vi "Measurement UI.vi"() -> ()   [LabVIEW 2021, in "Efficiency And Load Regulation_PMIC.lvlib"]
uses:
  Efficiency And Load Regulation_PMIC.lvlib
panel:
  in  "MeasGraphs":T1(tab)
  out "EfficiencyGraph":T2(graph)
  out "LoadRegulationGraph(V/A)":T2(graph)
  out "LoadRegulationGraph(%)":T2(graph)
  out "Maximum load regulation":dbl[](array[numeric])
  out "Minimum load regulation":dbl[](array[numeric])
  out "Maximum load voltage":dbl[](array[numeric])
  out "Minimum load voltage":dbl[](array[numeric])
  out "Maximum efficiency":dbl[](array[numeric])
  out "Minimum efficiency":dbl[](array[numeric])
  out "Source sweep points":i32
  out "Load voltage deviation":dbl[](array[numeric])
  out "Load voltages":dbl[](array[numeric])
  out "Voltage values":dbl[](array[numeric])
  out "Load sweep points":i32
  out "Efficiency":dbl[](array[numeric])
  out "Load currents":dbl[](array[numeric])
  in  "Source resource name":string caption="RESOURCE NAME"
  in  "Load resource name":string caption="RESOURCE NAME"
  out "MeasTable":string[][](table)
  out "Status":string
  in  "ELOADResourceName":refnum<k15> caption="RESOURCE NAME"
  in  "PPSResourceName":refnum<k15> caption="RESOURCE NAME"
  in  "Load sweep type":string(combo)="Logarithmic" caption="SWEEP TYPE"
  in  "DUT setup time":dbl=1.0 caption="DUT SETUP TIME" format="%#_6ps"
  in  "Source stop voltage":dbl=20.0 caption="STOP VOLTAGE" format="%#_6pV"
  in  "Source start voltage":dbl=6.0 caption="START VOLTAGE" format="%#_6pV"
  in  "Source voltage sweep points":i32=4 caption="NO. OF POINTS"
  in  "Aperture time":dbl=0.005 caption="APERTURE TIME" format="%#_6ps"
  in  "Source delay":dbl=0.005 caption="SOURCE DELAY" format="%#_6ps"
  in  "Load current sweep points/points per decade":i32=10 caption="PTS/PTS PER DECADE"
  in  "Load stop current":dbl=24.0 caption="STOP CURRENT" format="%#_6pA"
  in  "Load start current":dbl=0.1 caption="START CURRENT" format="%#_6pA"
  in  "Load voltage limit range":dbl=6.0 caption="VOLTAGE LIMIT RANGE" format="%#_6pV"
  in  "Source current limit":dbl=25.0 caption="CURRENT LIMIT" format="%#_6pA"
  in  "Source maximum power":dbl=300.0 caption="MAXIMUM POWER" format="%#_6pW"
  in  "Load configuration":string="Load configuration"
  in  "Source configuration":string="Source configuration"
  in  "Measurement settings":string="Measurement settings"
  in  "Nominal output voltage":dbl=3.3 caption="NOMINAL OUTPUT VOLTAGE" format="%#_6pV"
  in  "Mode of operation":T3(ring)=enum."Perform measurement" caption="MODE OF OPERATION"
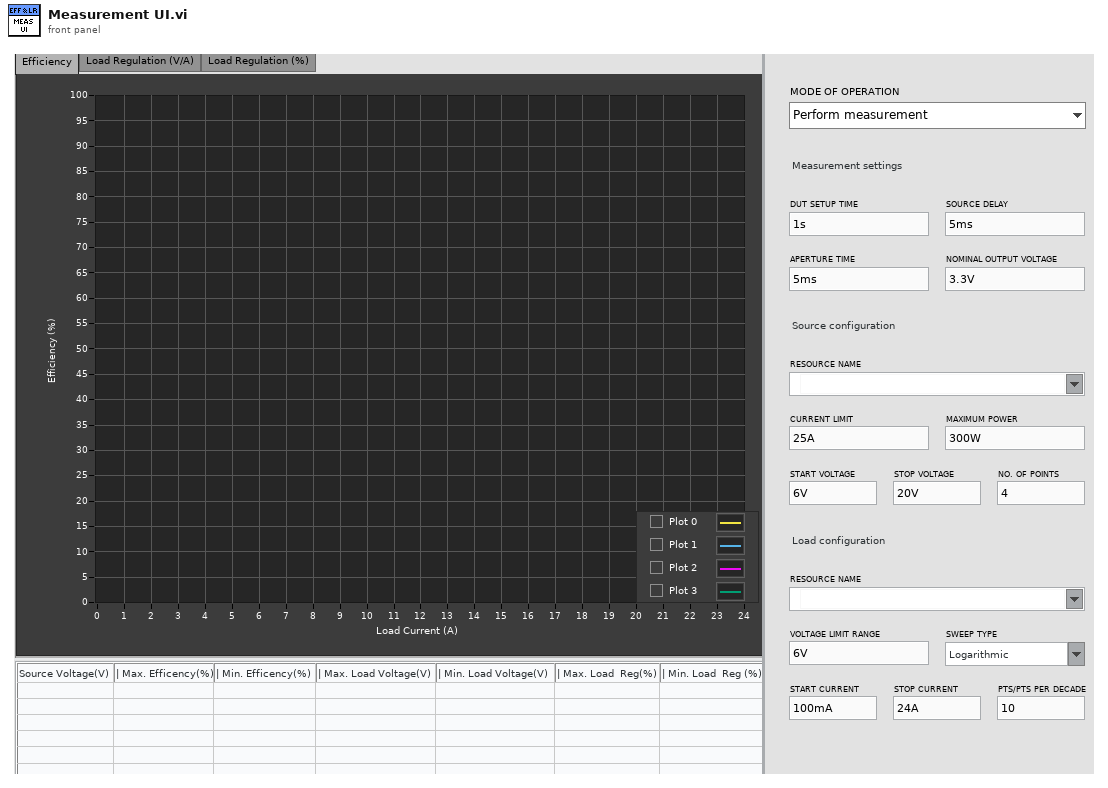
[diagram p1: front panel]
types:
  T1 = enum32{"Efficiency", "Load Regulation (V/A)", "Load Regulation (%)", "Hidden Controls"}
  T2 = cluster{"Load currents":dbl[], "Efficiency":dbl[]}[]
  T3 = enum32{"Power on the DUT", "Perform measurement", "Power off the DUT"}
  T4 = cluster{"Load currents":dbl[], "Efficiency":dbl[]}
  T5 = cluster{"Load currents":dbl[], "Load voltages":dbl[]}
  T6 = cluster{"Load currents":dbl[], "Load voltage deviation":dbl[]}
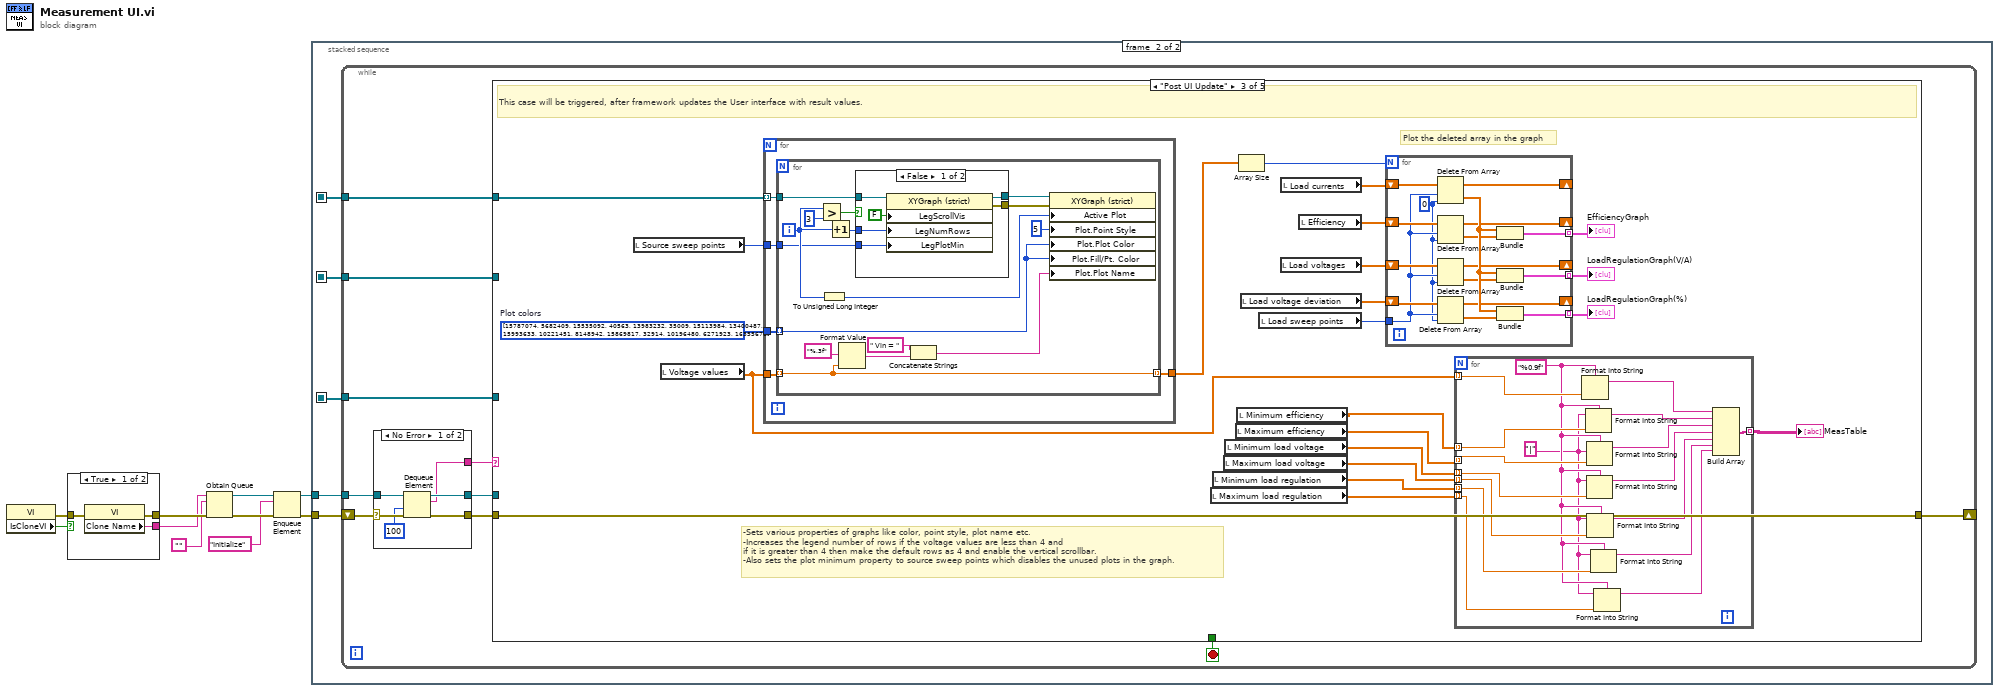
[diagram p0: block diagram]
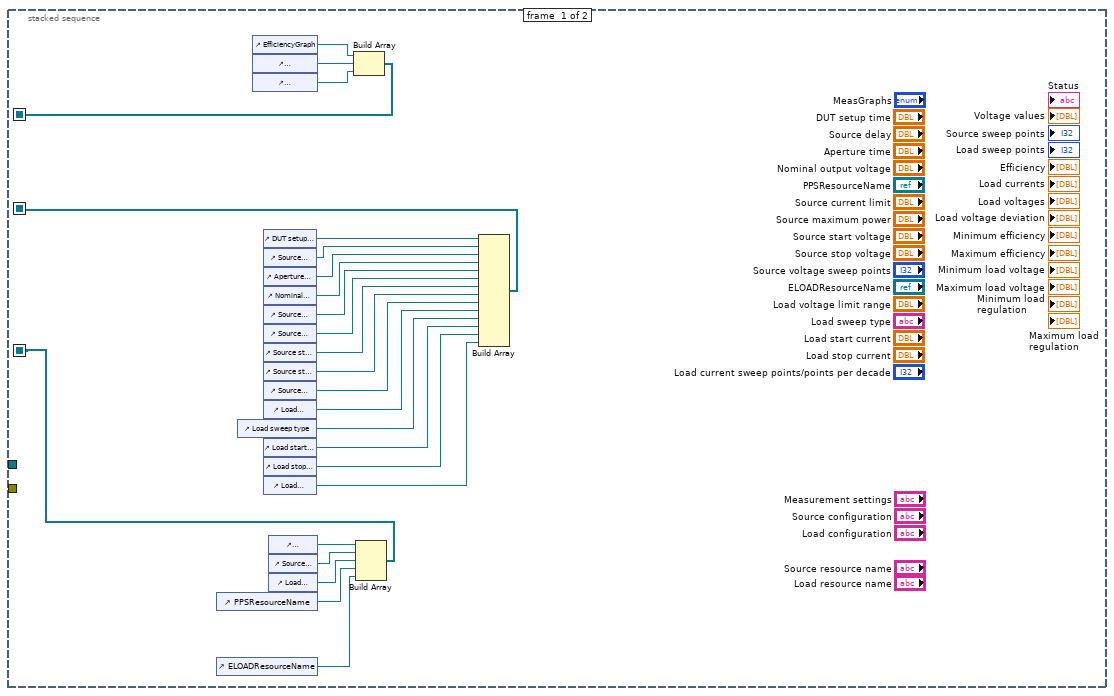
[diagram p2: hidden frame]
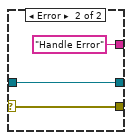
[diagram p3: hidden frame]
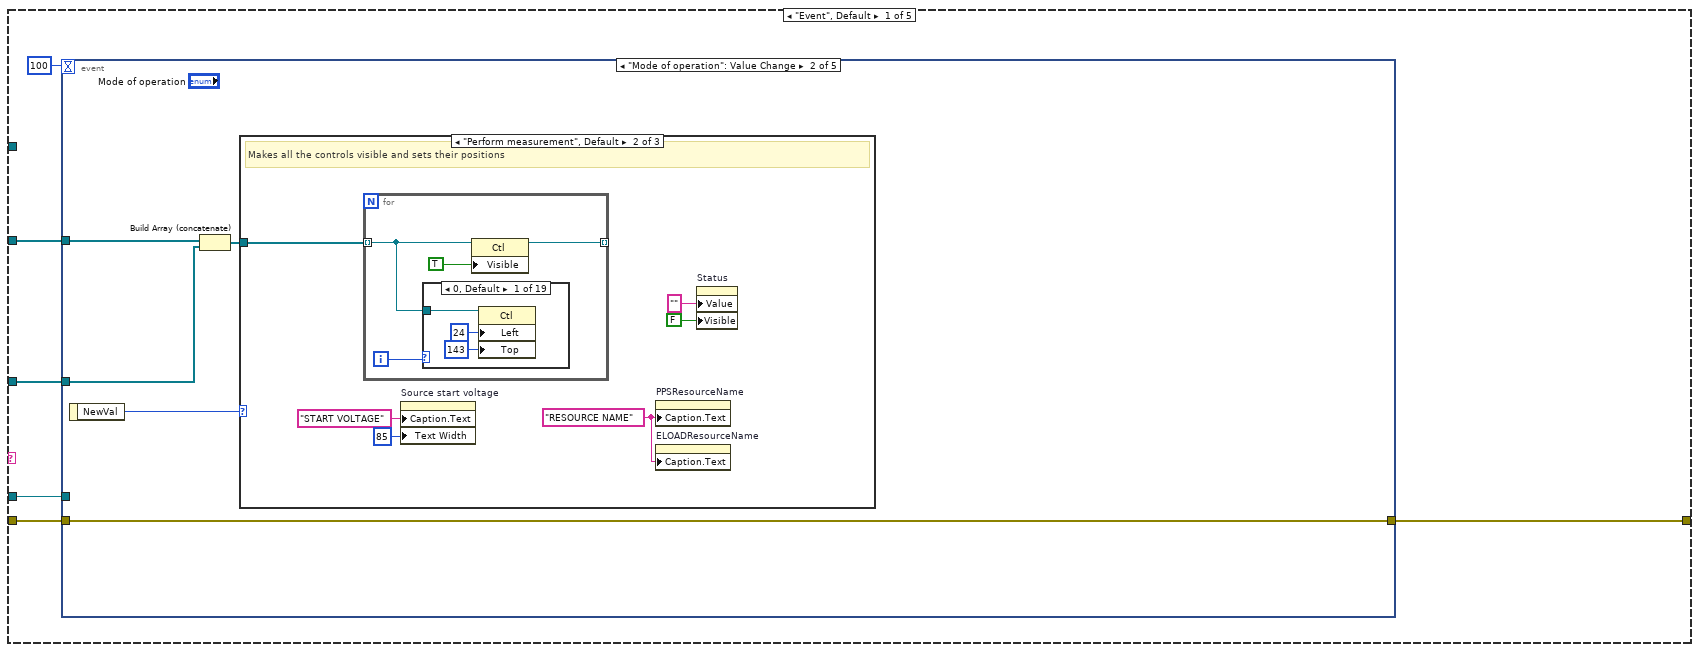
[diagram p4: hidden frame]
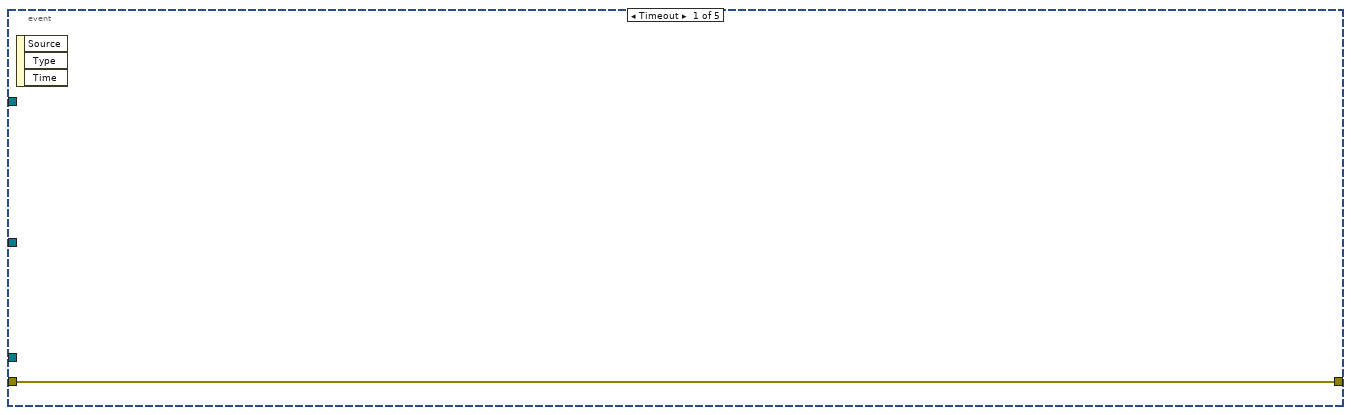
[diagram p5: hidden frame]
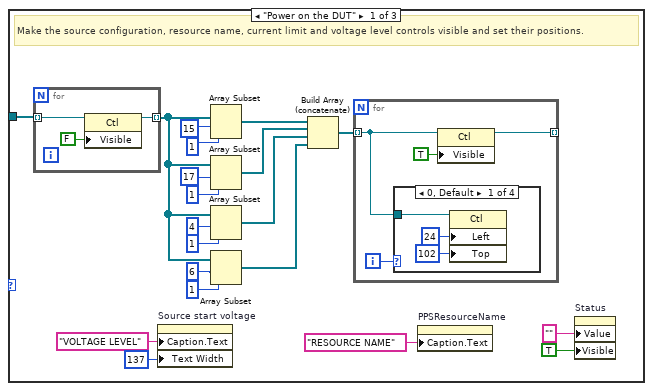
[diagram p6: hidden frame]
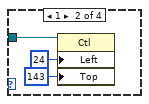
[diagram p7: hidden frame]
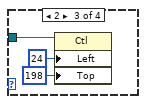
[diagram p8: hidden frame]
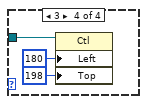
[diagram p9: hidden frame]
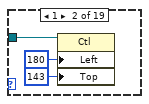
[diagram p10: hidden frame]
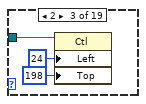
[diagram p11: hidden frame]
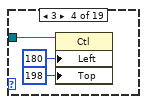
[diagram p12: hidden frame]
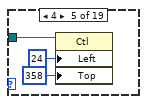
[diagram p13: hidden frame]
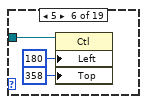
[diagram p14: hidden frame]
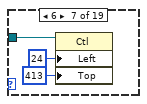
[diagram p15: hidden frame]
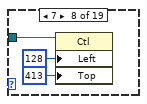
[diagram p16: hidden frame]
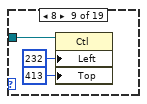
[diagram p17: hidden frame]
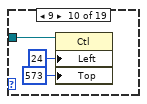
[diagram p18: hidden frame]
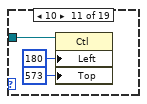
[diagram p19: hidden frame]
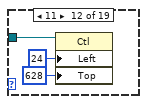
[diagram p20: hidden frame]
diagram:
  n1 = property class="VI"() -> (error out=w1:errorcluster, "IsCloneVI"=w2:bool)  [unwired: 2 in, 1 out]
  n2 = case shown="True" w2 {
    tunnel: [w13 w16] -> w10
    tunnel: [w12 w15] -> w9
    tunnel: w1 -> [w11 w14]
    frame True {
      n3 = property class="VI"(error in=w11) -> (error out=w13:errorcluster, "Clone Name"=w12:string)  [unwired: 1 in, 1 out]
    }
    frame False {
      n4 = property class="VI"(error in=w14) -> (error out=w16:errorcluster, "Name"=w15:string)  [unwired: 1 in, 1 out]
    }
  }
  n5 = Obtain Queue(name (unnamed)=w9, element data type="", error in (no error)=w10) -> (queue out=w6:refnum<queue>, error out=w8:errorcluster)  [unwired: 2 in, 1 out]
  n6 = Enqueue Element(queue=w6, element="Initialize", error in (no error)=w8) -> (queue out=w5:refnum<queue>, error out=w7:errorcluster)  [unwired: 1 in, 1 out]
  n7 = stacked-sequence {
    seq-local: [w17 _] -> [_ w44]
    seq-local: [w18 _] -> [_ w43]
    seq-local: [w19 _] -> [_ w42]
    tunnel: w7 -> [_ w46]
    tunnel: w5 -> [_ w45]
    frame #0 {
      n8 = control-ref of="PPSResourceName"() -> (w24:refnum<vi>)
      n9 = control-ref of="ELOADResourceName"() -> (w23:refnum<vi>)
      n10 = control-ref of="Load sweep type"() -> (w32:refnum<vi>)
      n11 = control-ref of="EfficiencyGraph"() -> (w22:refnum<vi>)
      n12 = control-ref of="LoadRegulationGraph(V/A)"() -> (w21:refnum<vi>)
      n13 = control-ref of="LoadRegulationGraph(%)"() -> (w20:refnum<vi>)
      n14 = control-ref of="DUT setup time"() -> (w41:refnum<vi>)
      n15 = control-ref of="Source delay"() -> (w40:refnum<vi>)
      n16 = control-ref of="Aperture time"() -> (w39:refnum<vi>)
      n17 = control-ref of="Nominal output voltage"() -> (w28:refnum<vi>)
      n18 = control-ref of="Source current limit"() -> (w38:refnum<vi>)
      n19 = control-ref of="Source maximum power"() -> (w37:refnum<vi>)
      n20 = control-ref of="Source start voltage"() -> (w36:refnum<vi>)
      n21 = control-ref of="Source stop voltage"() -> (w35:refnum<vi>)
      n22 = control-ref of="Source voltage sweep points"() -> (w34:refnum<vi>)
      n23 = control-ref of="Load voltage limit range"() -> (w33:refnum<vi>)
      n24 = control-ref of="Load start current"() -> (w31:refnum<vi>)
      n25 = control-ref of="Load stop current"() -> (w30:refnum<vi>)
      n26 = control-ref of="Load current sweep points/points per decade"() -> (w29:refnum<vi>)
      n27 = control-ref of="Measurement settings"() -> (w27:refnum<vi>)
      n28 = control-ref of="Source configuration"() -> (w25:refnum<vi>)
      n29 = control-ref of="Load configuration"() -> (w26:refnum<vi>)
      n30 = Build Array(w22, w21, w20) -> (w17:refnum<vi>[])
      n31 = Build Array(w27, w25, w26, w24, w23) -> (w19:refnum<vi>[])
      n32 = Build Array(w41, w40, w39, w28, w38, w37, w36, w35, w34, w33, w32, w31, w30, w29) -> (w18:refnum<vi>[])
    }
    frame #1 {
      n33 = while {
        shift-right: [w51] -> _
        shift-left: w46 -> [w56]
        tunnel: w45 -> [w54]
        tunnel: w43 -> [w49]
        tunnel: w42 -> [w48]
        tunnel: w44 -> [w47]
        stop <- w50 stop-if-true
        n34 = case shown="No Error" w56 {
          selector: w56 -> [w62 w65]
          tunnel: [w61 w65] -> w55
          tunnel: w54 -> [w60 w64]
          tunnel: [w59 w64] -> w53
          tunnel: [w58 "Handle Error"] -> w52
          frame No Error {
            n35 = Dequeue Element(queue=w60, timeout in ms (-1)=100, error in (no error)=w62) -> (queue out=w59:refnum<queue>, element=w58:string, error out=w61:errorcluster)  [unwired: 1 out]
          }
          frame Error {
          }
        }
        n36 = case shown="\"Post UI Update\"" w52 {
          tunnel: w55 -> [w70 w218 w242 w322 w323]
          tunnel: w53 -> [w68 _ _ w320 _]
          tunnel: [w71 w218 w242 w314 w323] -> w51
          tunnel: [_ _ _ TRUE _] -> w50
          tunnel: w49 -> [w67 _ _ w312 _]
          tunnel: w48 -> [w66 _ _ w311 _]
          tunnel: w47 -> [_ w217 w232 w313 _]
          frame "Event", Default {
            n37 = event shown="[1] \"Mode of operation\": Value Change" {
              selector: _ -> [_ _ _ _ _]
              dyn-events: _ -> [_ _ _ _ _]
              timeout: 100 -> [_ _ _ _ _]
              tunnel: [w72 w73 w206 w208 w212] -> w71
              tunnel: w70 -> [w72 w73 w206 w208 w213]
              tunnel: w68 -> [_ _ _ _ w211]
              tunnel: w67 -> [_ w74 _ _ _]
              tunnel: w66 -> [_ w76 _ _ _]
              event Timeout {
                n38 = event-data() -> ()  [unwired: 1 in, 3 out]
              }
              event "Mode of operation": Value Change {
                n39 = event-data() -> ("NewVal"=w77:T3)  [unwired: 1 in]
                n40 = Build Array (concatenate)(w74, w76) -> (w75:refnum<vi>[])
                n41 = case shown="\"Perform measurement\", Default" w77 {
                  tunnel: w75 -> [w89 w122 w189]
                  frame "Power on the DUT" {
                    # "Make the source configuration, resource name, current limit and voltage level controls visible and set their positions."
                    n42 = for {
                      tunnel: w89 -> [w100] mode=indexing
                      tunnel: [w98] -> w86 mode=indexing
                      n43 = property class="Ctl"(reference=w100, "Visible"=FALSE) -> (reference out=w98:refnum<vi>)  [unwired: 1 in, 1 out]
                    }
                    n44 = property on="Source start voltage" class="DigNum (strict)"("Caption.Text"="VOLTAGE LEVEL", "Text Width"=u32 137) -> ()  [unwired: 2 in, 2 out]
                    n45 = Array Subset(array=w86, index=15 ("length"), length=1 ("index")) -> (w88:refnum<vi>[])
                    n46 = Array Subset(array=w86, index=17 ("length"), length=1 ("index")) -> (w87:refnum<vi>[])
                    n47 = Array Subset(array=w86, index=4 ("length"), length=1 ("index")) -> (w85:refnum<vi>[])
                    n48 = Array Subset(array=w86, index=6 ("length"), length=1 ("index")) -> (w83:refnum<vi>[])
                    n49 = Build Array (concatenate)(w88, w87, w85, w83) -> (w84:refnum<vi>[])
                    n50 = for {
                      tunnel: [w103] -> _ mode=indexing
                      tunnel: w84 -> [w101] mode=indexing
                      i -> [w102]
                      n51 = case shown="0, Default" w102 {
                        tunnel: w101 -> [w107 w110 w113 w116]
                        frame 0, Default {
                          n52 = property class="Ctl"(reference=w107, "Left"=24 ("Position:Left"), "Top"=102 ("Position:Top")) -> ()  [unwired: 1 in, 2 out]
                        }
                        frame 1 {
                          n53 = property class="Ctl"(reference=w110, "Left"=24 ("Position:Left"), "Top"=143 ("Position:Top")) -> ()  [unwired: 1 in, 2 out]
                        }
                        frame 2 {
                          n54 = property class="Ctl"(reference=w113, "Left"=24 ("Position:Left"), "Top"=198 ("Position:Top")) -> ()  [unwired: 1 in, 2 out]
                        }
                        frame 3 {
                          n55 = property class="Ctl"(reference=w116, "Left"=180 ("Position:Left"), "Top"=198 ("Position:Top")) -> ()  [unwired: 1 in, 2 out]
                        }
                      }
                      n56 = property class="Ctl"(reference=w101, "Visible"=TRUE) -> (reference out=w103:refnum<vi>)  [unwired: 1 in, 1 out]
                    }
                    n57 = property on="PPSResourceName" class="IVIName"("Caption.Text"="RESOURCE NAME") -> ()  [unwired: 2 in, 2 out]
                    n58 = property on="Status" class="Str"("Value"="" ("Status"), "Visible"=TRUE) -> ()  [unwired: 2 in, 2 out]
                  }
                  frame "Perform measurement", Default {
                    w120 = "RESOURCE NAME" ("Caption.Text")
                    # "Makes all the controls visible and sets their positions"
                    n59 = for {
                      tunnel: w122 -> [w123] mode=indexing
                      tunnel: [w125] -> _ mode=indexing
                      i -> [w124]
                      n60 = case shown="0, Default" w124 {
                        tunnel: w123 -> [w129 w132 w135 w138 w141 w144 w147 w150 w153 w156 w159 w162 w165 w168 w171 w174 w177 w180 w183]
                        frame 0, Default {
                          n61 = property class="Ctl"(reference=w129, "Left"=24 ("Position:Left"), "Top"=143 ("Position:Top")) -> ()  [unwired: 1 in, 2 out]
                        }
                        frame 1 {
                          n62 = property class="Ctl"(reference=w132, "Left"=180 ("Position:Left"), "Top"=143 ("Position:Top")) -> ()  [unwired: 1 in, 2 out]
                        }
                        frame 2 {
                          n63 = property class="Ctl"(reference=w135, "Left"=24 ("Position:Left"), "Top"=198 ("Position:Top")) -> ()  [unwired: 1 in, 2 out]
                        }
                        frame 3 {
                          n64 = property class="Ctl"(reference=w138, "Left"=180 ("Position:Left"), "Top"=198 ("Position:Top")) -> ()  [unwired: 1 in, 2 out]
                        }
                        frame 4 {
                          n65 = property class="Ctl"(reference=w141, "Left"=24 ("Position:Left"), "Top"=358 ("Position:Top")) -> ()  [unwired: 1 in, 2 out]
                        }
                        frame 5 {
                          n66 = property class="Ctl"(reference=w144, "Left"=180 ("Position:Left"), "Top"=358 ("Position:Top")) -> ()  [unwired: 1 in, 2 out]
                        }
                        frame 6 {
                          n67 = property class="Ctl"(reference=w147, "Left"=24 ("Position:Left"), "Top"=413 ("Position:Top")) -> ()  [unwired: 1 in, 2 out]
                        }
                        frame 7 {
                          n68 = property class="Ctl"(reference=w150, "Left"=128 ("Position:Left"), "Top"=413 ("Position:Top")) -> ()  [unwired: 1 in, 2 out]
                        }
                        frame 8 {
                          n69 = property class="Ctl"(reference=w153, "Left"=232 ("Position:Left"), "Top"=413 ("Position:Top")) -> ()  [unwired: 1 in, 2 out]
                        }
                        frame 9 {
                          n70 = property class="Ctl"(reference=w156, "Left"=24 ("Position:Left"), "Top"=573 ("Position:Top")) -> ()  [unwired: 1 in, 2 out]
                        }
                        frame 10 {
                          n71 = property class="Ctl"(reference=w159, "Left"=180 ("Position:Left"), "Top"=573 ("Position:Top")) -> ()  [unwired: 1 in, 2 out]
                        }
                        frame 11 {
                          n72 = property class="Ctl"(reference=w162, "Left"=24 ("Position:Left"), "Top"=628 ("Position:Top")) -> ()  [unwired: 1 in, 2 out]
                        }
                        frame 12 {
                          n73 = property class="Ctl"(reference=w165, "Left"=128 ("Position:Left"), "Top"=628 ("Position:Top")) -> ()  [unwired: 1 in, 2 out]
                        }
                        frame 13 {
                          n74 = property class="Ctl"(reference=w168, "Left"=232 ("Position:Left"), "Top"=628 ("Position:Top")) -> ()  [unwired: 1 in, 2 out]
                        }
                        frame 14 {
                          n75 = property class="Ctl"(reference=w171, "Left"=24 ("Position:Left"), "Top"=102 ("Position:Top")) -> ()  [unwired: 1 in, 2 out]
                        }
                        frame 15 {
                          n76 = property class="Ctl"(reference=w174, "Left"=24 ("Position:Left"), "Top"=262 ("Position:Top")) -> ()  [unwired: 1 in, 2 out]
                        }
                        frame 16 {
                          n77 = property class="Ctl"(reference=w177, "Left"=24 ("Position:Left"), "Top"=477 ("Position:Top")) -> ()  [unwired: 1 in, 2 out]
                        }
                        frame 17 {
                          n78 = property class="Ctl"(reference=w180, "Left"=24 ("Position:Left"), "Top"=303 ("Position:Top")) -> ()  [unwired: 1 in, 2 out]
                        }
                        frame 18 {
                          n79 = property class="Ctl"(reference=w183, "Left"=24 ("Position:Left"), "Top"=518 ("Position:Top")) -> ()  [unwired: 1 in, 2 out]
                        }
                      }
                      n80 = property class="Ctl"(reference=w123, "Visible"=TRUE) -> (reference out=w125:refnum<vi>)  [unwired: 1 in, 1 out]
                    }
                    n81 = property on="Source start voltage" class="DigNum (strict)"("Caption.Text"="START VOLTAGE", "Text Width"=u32 85) -> ()  [unwired: 2 in, 2 out]
                    n82 = property on="PPSResourceName" class="IVIName"("Caption.Text"=w120) -> ()  [unwired: 2 in, 2 out]
                    n83 = property on="ELOADResourceName" class="IVIName"("Caption.Text"=w120) -> ()  [unwired: 2 in, 2 out]
                    n84 = property on="Status" class="Str"("Value"="" ("Status"), "Visible"=FALSE) -> ()  [unwired: 2 in, 2 out]
                  }
                  frame "Power off the DUT" {
                    # "Makes only the Source and Load Resource Name controls visible and sets their positions"
                    n85 = for {
                      tunnel: w189 -> [w194] mode=indexing
                      tunnel: [w193] -> w188 mode=indexing
                      n86 = property class="Ctl"(reference=w194, "Visible"=FALSE) -> (reference out=w193:refnum<vi>)  [unwired: 1 in, 1 out]
                    }
                    n87 = Array Subset(array=w188, index=17 ("length"), length=2 ("index")) -> (w190:refnum<vi>[])
                    n88 = property on="PPSResourceName" class="IVIName"("Caption.Text"="SOURCE RESOURCE NAME") -> ()  [unwired: 2 in, 2 out]
                    n89 = property on="ELOADResourceName" class="IVIName"("Caption.Text"="LOAD RESOURCE NAME") -> ()  [unwired: 2 in, 2 out]
                    n90 = for {
                      tunnel: w190 -> [w196] mode=indexing
                      tunnel: [w198] -> _ mode=indexing
                      i -> [w197]
                      n91 = case shown="0, Default" w197 {
                        tunnel: w196 -> [w202 w205]
                        frame 0, Default {
                          n92 = property class="Ctl"(reference=w202, "Left"=24 ("Position:Left"), "Top"=102 ("Position:Top")) -> ()  [unwired: 1 in, 2 out]
                        }
                        frame 1 {
                          n93 = property class="Ctl"(reference=w205, "Left"=24 ("Position:Left"), "Top"=157 ("Position:Top")) -> ()  [unwired: 1 in, 2 out]
                        }
                      }
                      n94 = property class="Ctl"(reference=w196, "Visible"=TRUE) -> (reference out=w198:refnum<vi>)  [unwired: 1 in, 1 out]
                    }
                    n95 = property on="Status" class="Str"("Value"="" ("Status"), "Visible"=TRUE) -> ()  [unwired: 2 in, 2 out]
                  }
                }
              }
              event "PPSResourceName": Value Change {
                n96 = event-data() -> ()  [unwired: 1 in, 1 out]
                n97 = property on="PPSResourceName" class="IVIName"() -> ("Value"=w207:refnum<k15>)  [unwired: 2 in, 2 out]
                n98 = property on="Source resource name" class="Str"("Value"=w207) -> ()  [unwired: 2 in, 2 out]
              }
              event "ELOADResourceName": Value Change {
                n99 = event-data() -> ()  [unwired: 1 in, 1 out]
                n100 = property on="ELOADResourceName" class="IVIName"() -> ("Value"=w209:refnum<k15>)  [unwired: 2 in, 2 out]
                n101 = property on="Load resource name" class="Str"("Value"=w209) -> ()  [unwired: 2 in, 2 out]
              }
              event Panel Close? {
                n102 = event-data() -> ()  [unwired: 1 in, 4 out]
                n103 = Enqueue Element(queue=w211, element="Exit", error in (no error)=w213) -> (error out=w212:errorcluster)  [unwired: 1 in, 2 out]
                n104 = event-data("Discard?"=TRUE) -> ()  [unwired: 1 in, 1 out]
              }
            }
          }
          frame "Initialize" {
            w216 = "<Select Device>"
            n105 = for {
              tunnel: w217 -> [w219] mode=indexing
              n106 = property class="XYGraph (strict)"(reference=w219, "ActPaletteTool"=2 ("Palette:Active Tool")) -> ()  [unwired: 1 in, 2 out]
            }
            n107 = property on="PPSResourceName" class="IVIName"("Value"=w216) -> ()  [unwired: 2 in, 2 out]
            n108 = property on="ELOADResourceName" class="IVIName"("Value"=w216) -> ()  [unwired: 2 in, 2 out]
            n109 = property on="Status" class="Str"("Visible"=FALSE) -> ()  [unwired: 2 in, 2 out]
          }
          frame "Post UI Update" {
            w231 = u32[] [15787074, 5682409, 15535092, 40563, 13983232, 35009, 15113984, 13400487, 15993633, 10221451, 8148942, 15869817, 32914, 10196480, 6271923, 16355671]  # Plot colors
            # "-Sets various properties of graphs like color, point style, plot name etc.\n-Increases the legend number of rows if the voltage values are less than 4 and \nif it is greater than 4 then make the default rows as 4 and enable the vertical scrollbar.\n-Also sets the plot minimum property to source sweep points which disables the unused plots in the graph."
            # "Plot the deleted array in the graph"
            # "This case will be triggered, after framework updates the User interface with result values."
            n110 = local read "Source sweep points"() -> (w230:i32)
            n111 = local read "Voltage values"() -> (w227:dbl[])
            n112 = for {
              tunnel: w227 -> [w264]
              tunnel: [w263] -> w229
              tunnel: w232 -> [w262] mode=indexing
              tunnel: w230 -> [w261]
              tunnel: w231 -> [w260]
              n113 = for {
                tunnel: w264 -> [w277] mode=indexing
                tunnel: [w277] -> w263 mode=indexing
                tunnel: w262 -> [w270]
                tunnel: w261 -> [w267]
                tunnel: w260 -> [w273] mode=indexing
                i -> [w271]
                n114 = Greater?(x=w271, y=3) -> (0:w275:bool)
                n115 = To Unsigned Long Integer(number=w271) -> (unsigned 32bit integer=w274:u32)
                n116 = Increment(x=w271) -> (x+1=w269:i32)
                n117 = Format Value(format string="%.3f", value (0)=w277) -> (output string=w280:string)  [unwired: 1 out]
                n118 = case shown="False" w275 {
                  tunnel: w270 -> [w286 w292]
                  tunnel: w269 -> [w285 _]
                  tunnel: [w284 w291] -> w268
                  tunnel: w267 -> [w282 w287]
                  tunnel: [w283 w290] -> w266
                  frame False {
                    n119 = property on="Property Node" class="XYGraph (strict)"(reference=w286, "LegScrollVis"=FALSE ("Legend:Scrollbar Visible"), "LegNumRows"=w285, "LegPlotMin"=w282) -> (reference out=w284:refnum<vi>, error out=w283:errorcluster)  [unwired: 1 in]
                  }
                  frame True {
                    n120 = property on="Property Node" class="XYGraph (strict)"(reference=w292, "LegScrollVis"=TRUE ("Legend:Scrollbar Visible"), "LegNumRows"=u32 4 ("Legend:Number of Rows"), "LegPlotMin"=w287) -> (reference out=w291:refnum<vi>, error out=w290:errorcluster)  [unwired: 1 in]
                  }
                }
                n121 = Concatenate Strings(" Vin = " ("string"), w280) -> (w265:string)
                n122 = property on="Property Node" class="XYGraph (strict)"(reference=w268, error in=w266, "Active Plot"=w274, "Plot.Point Style"=u8 5, "Plot.Plot Color"=w273, "Plot.Fill/Pt. Color"=w273, "Plot.Plot Name"=w265) -> ()  [unwired: 2 out]
              }
            }
            n123 = local read "Maximum load regulation"() -> (w222:dbl[])
            n124 = local read "Minimum load regulation"() -> (w223:dbl[])
            n125 = local read "Maximum load voltage"() -> (w224:dbl[])
            n126 = local read "Minimum load voltage"() -> (w225:dbl[])
            n127 = local read "Maximum efficiency"() -> (w226:dbl[])
            n128 = local read "Minimum efficiency"() -> (w228:dbl[])
            n129 = Array Size(array=w229) -> (size(s)=w239:i32)
            n130 = local read "Load voltage deviation"() -> (w241:dbl[])
            n131 = local read "Load sweep points"() -> (w236:i32)
            n132 = local read "Load voltages"() -> (w240:dbl[])
            n133 = local read "Load currents"() -> (w238:dbl[])
            n134 = local read "Efficiency"() -> (w237:dbl[])
            n135 = for {
              N: w239 -> [_]
              tunnel: [w309] -> w233 mode=indexing
              tunnel: [w308] -> w234 mode=indexing
              tunnel: [w307] -> w235 mode=indexing
              tunnel: w236 -> [w294]
              shift-right: [w302] -> _
              shift-left: w238 -> [w306]
              shift-right: [w300] -> _
              shift-left: w237 -> [w305]
              shift-right: [w299] -> _
              shift-left: w240 -> [w304]
              shift-right: [w298] -> _
              shift-left: w241 -> [w303]
              w293 = 0 ("index")
              n136 = Delete From Array(array=w306, length=w294, index=w293) -> (deleted portion=w301:dbl[], array with subset deleted=w302:dbl[])
              n137 = Delete From Array(array=w305, length=w294, index=w293) -> (deleted portion=w295:dbl[], array with subset deleted=w300:dbl[])
              n138 = Delete From Array(array=w304, length=w294, index=w293) -> (deleted portion=w296:dbl[], array with subset deleted=w299:dbl[])
              n139 = Delete From Array(array=w303, length=w294, index=w293) -> (deleted portion=w297:dbl[], array with subset deleted=w298:dbl[])
              n140 = Bundle("Load currents"=w301, "Efficiency"=w295) -> (w309:T4)  [unwired: 1 in]
              n141 = Bundle("Load currents"=w301, "Load voltages"=w296) -> (w308:T5)  [unwired: 1 in]
              n142 = Bundle("Load currents"=w301, "Load voltage deviation"=w297) -> (w307:T6)  [unwired: 1 in]
            }
            "EfficiencyGraph" <- w233
            "LoadRegulationGraph(V/A)" <- w234
            "LoadRegulationGraph(%)" <- w235
            n143 = for {
              tunnel: w225 -> [w255] mode=indexing
              tunnel: w228 -> [w257] mode=indexing
              tunnel: [w258] -> w221 mode=indexing
              tunnel: w226 -> [w256] mode=indexing
              tunnel: w224 -> [w254] mode=indexing
              tunnel: w223 -> [w253] mode=indexing
              tunnel: w227 -> [w249] mode=indexing
              tunnel: w222 -> [w244] mode=indexing
              w246 = "%0.9f" ("initial string")
              w245 = "|" ("initial string")
              n144 = Format Into String(format string=w246, w249) -> (resulting string=w248:string)  [unwired: 2 in, 1 out]
              n145 = Format Into String(format string=w246, initial string=w245, w257) -> (resulting string=w259:string)  [unwired: 1 in, 1 out]
              n146 = Format Into String(format string=w246, initial string=w245, w256) -> (resulting string=w252:string)  [unwired: 1 in, 1 out]
              n147 = Format Into String(format string=w246, initial string=w245, w255) -> (resulting string=w251:string)  [unwired: 1 in, 1 out]
              n148 = Format Into String(format string=w246, initial string=w245, w254) -> (resulting string=w250:string)  [unwired: 1 in, 1 out]
              n149 = Format Into String(format string=w246, initial string=w245, w253) -> (resulting string=w247:string)  [unwired: 1 in, 1 out]
              n150 = Format Into String(format string=w246, initial string=w245, w244) -> (resulting string=w243:string)  [unwired: 1 in, 1 out]
              n151 = Build Array(w248, w259, w252, w251, w250, w247, w243) -> (w258:string[])
            }
            "MeasTable" <- w221
          }
          frame "Exit" {
            # "This case is triggered to close the User Interface from framework"
            n152 = Build Array (concatenate)(w313, w312, w311) -> (w310:refnum<vi>[])
            n153 = Close Reference(reference=w310) -> (error out=w316:errorcluster)  [unwired: 1 in]
            n154 = Flush Queue(queue=w320, error in (no error)=w322) -> (queue out=w319:refnum<queue>, error out=w318:errorcluster)  [unwired: 1 out]
            n155 = Release Queue(queue=w319, force destroy? (F)=TRUE, error in (no error)=w318) -> (error out=w315:errorcluster)  [unwired: 2 out]
            n156 = Merge Errors(w316, w315) -> (w314:errorcluster)
          }
          frame "Handle Error" {
          }
        }
      }
    }
  }
